vi "Draw_Cage_Outline_(t-maze).vi"(0 "Picture refnum in":T1, 1 "Bounding rectangle for cage outline, pix":T2, 2 "Background color":u32(colorbox), 3 "Error In":errorcluster, 4 "Inner donut scale factor":dbl=0.56 format="%#_13g") -> (5 "Picture refnum out":T1, 7 "Error Out":errorcluster)   [LabVIEW 2018, in "Cage Diagram.lvlib"]
uses:
  Cage Diagram.lvlib
  <vilib>/vision/Image Controls.llb/IMAQ Image.ctl
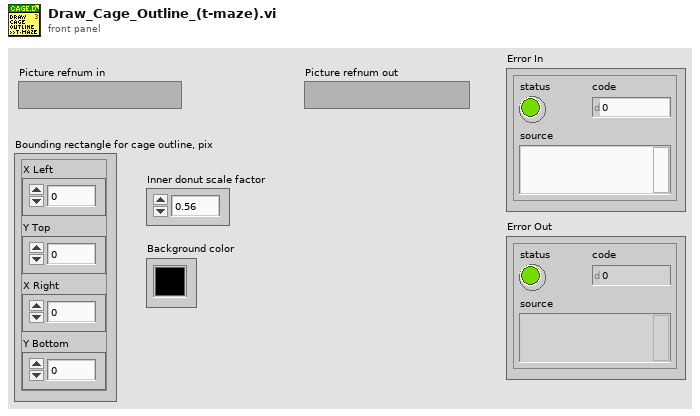
[diagram p1: front panel]
types:
  T1 = typedef "IMAQ Image.ctl" = refnum<image>
  T2 = cluster{"X Left":i32, "Y Top":i32, "X Right":i32, "Y Bottom":i32}
  T3 = cluster{"X Left":dbl, "Y Top":dbl, "X Right":dbl, "Y Bottom":dbl}
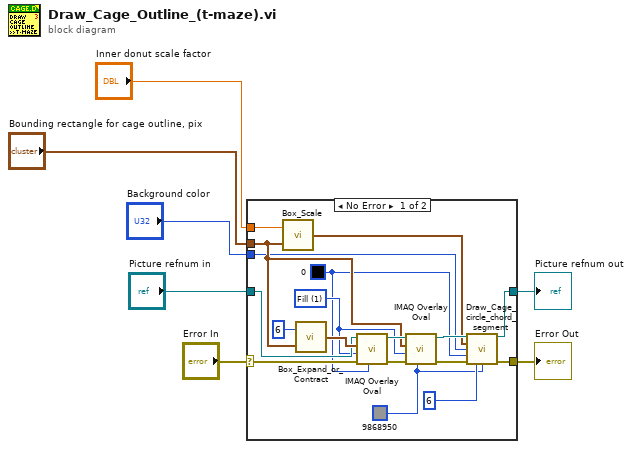
[diagram p0: block diagram]
diagram:
  n1 = case shown="No Error" "Error In" {
    selector: "Error In" -> [w23 w26]
    tunnel: [w15 w27] -> w6
    tunnel: "Picture refnum in" -> [w24 w27]
    tunnel: "Bounding rectangle for cage outline, pix" -> [w19 _]
    tunnel: [w16 w26] -> w3
    tunnel: "Background color" -> [w9 _]
    tunnel: "Inner donut scale factor" -> [w18 _]
    frame No Error {
      w8 = u32 9868950 ("Color")
      w10 = u32 0 ("Color")
      w17 = u32 1 items=["Frame", "Fill"] ("Drawing Mode (Frame)")
      n2 = call "Box_Scale.vi"("Rectangle in"=w19, "Scale factor"=w18) -> ("Rectangle out"=w12:T3)
      n3 = call "Box_Expand_or_Contract.vi"("Rectangle in"=w19, "Expand/Contract"=6) -> ("Rectangle out"=w25:T3)
      n4 = call "IMAQ Overlay Oval"("Color"=w10, "error in (no error)"=w23, "Drawing Mode (Frame)"=w17, "Bounding Rectangle"=w25, "Image"=w24) -> ("error out"=w21:errorcluster, "Image Out"=w22:T1)  [unwired: 5 in]
      n5 = call "IMAQ Overlay Oval"("Color"=w8, "error in (no error)"=w21, "Drawing Mode (Frame)"=w17, "Bounding Rectangle"=w19, "Image"=w22) -> ("error out"=w14:errorcluster, "Image Out"=w13:T1)  [unwired: 5 in]
      n6 = call "Draw_Cage_circle_chord_segment.vi"("Picture refnum in"=w13, "Bounding rectangle in"=w12, "Fill color"=w9, "Outline color"=w10, "Error In"=w14, "Border thickness, pix"=6, "Cage floor color"=w8) -> ("Picture refnum out"=w15:T1, "Error Out"=w16:errorcluster)  [unwired: 6 in, 1 out]
    }
    frame Error {
    }
  }
  "Error Out" <- w3
  "Picture refnum out" <- w6
